vi "Delete Config.vi"(8 "error in (no error)":errorcluster, 9 "Config Selected":string, 10 "Config Select Ref":refnum<vi>, 11 "GUI in":refnum<class "GUI.lvclass">) -> (0 "error out":errorcluster, 3 "GUI out":refnum<class "GUI.lvclass">)   [LabVIEW 2020, in "GUI.lvlib" / "GUI.lvclass"]
uses:
  GUI.lvclass
  GUI.lvclass/GUI.ctl
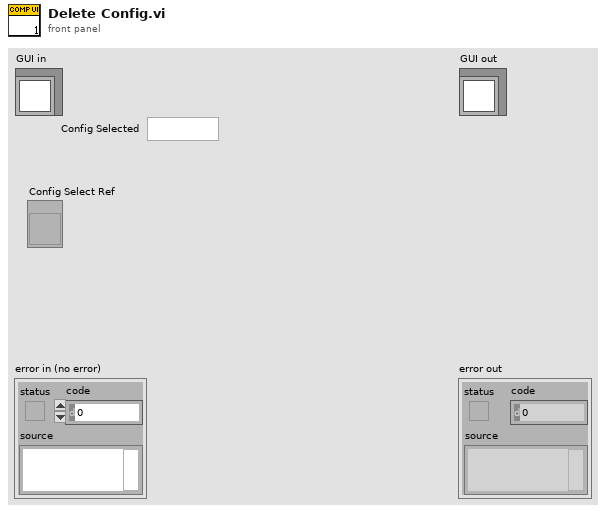
[diagram p1: front panel]
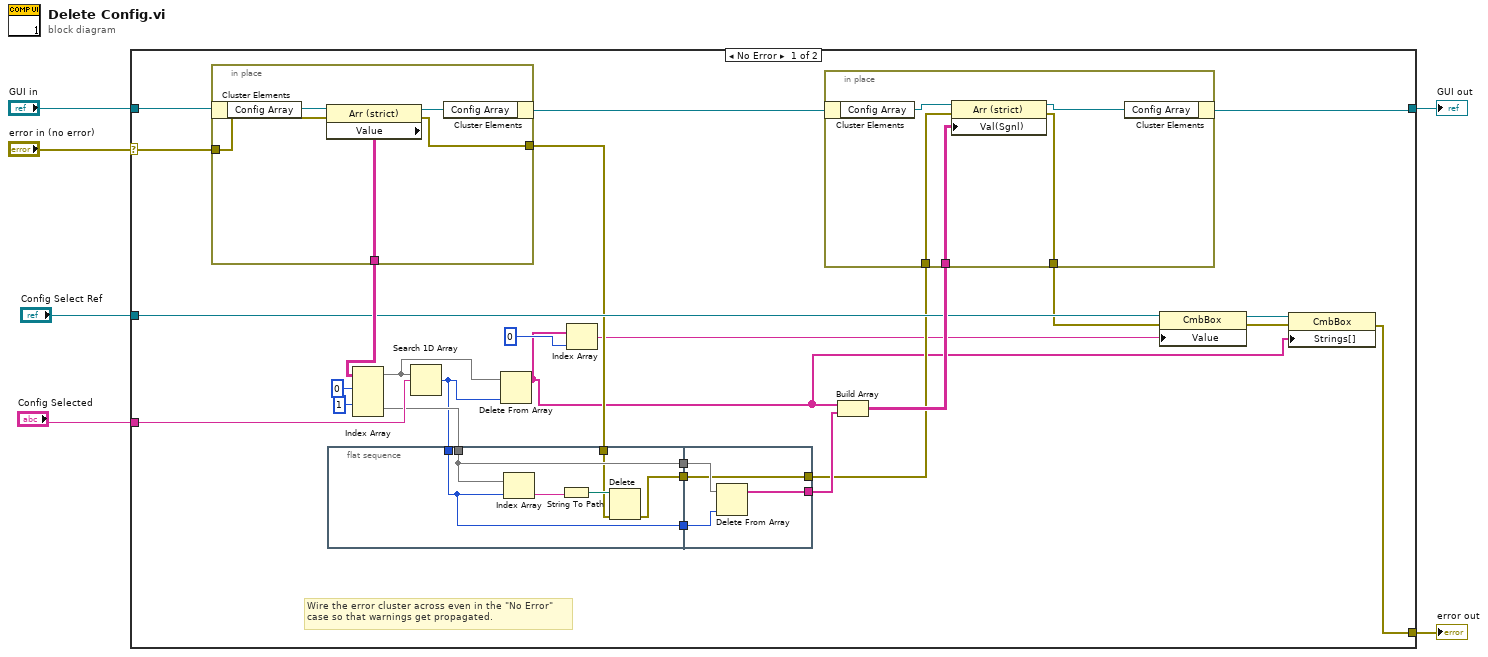
[diagram p0: block diagram]
diagram:
  n1 = case shown="No Error" "error in (no error)" {
    selector: "error in (no error)" -> [w18 w54]
    tunnel: [w9 w54] -> w5
    tunnel: [w21 w53] -> w3
    tunnel: "GUI in" -> [w32 w53]
    tunnel: "Config Selected" -> [w28 _]
    tunnel: "Config Select Ref" -> [w19 _]
    frame No Error {
      # "Wire the error cluster across even in the \"No Error\"\ncase so that warnings get propagated."
      n2 = in-place {
        in-place-border: [w51] -> w29
        in-place-border: w18 -> [w49]
        in-place-border: [w48] -> w17
        n3 = in-place-cluster #1(w32) -> ("Config Array"=w52:refnum<vi>)
        n4 = property class="Arr (strict)"(reference=w52, error in=w49) -> (reference out=w50:refnum<vi>, error out=w48:errorcluster, "Value"=w51:string[][])
        n5 = in-place-cluster #1("Config Array"=w50) -> (w22:refnum<class "GUI.lvclass">)
      }
      n6 = flat-sequence {
        tunnel: w26 -> [w41]
        tunnel: w7 -> [w40]
        tunnel: [w41] -> w25
        tunnel: [w40] -> w24
        tunnel: w17 -> [w39]
        tunnel: [w38] -> w16
        tunnel: w25 -> [w47]
        tunnel: w24 -> [w46]
        tunnel: [w45] -> w23
        tunnel: [w44] -> w15
        tunnel: w16 -> [w44]
        frame #0 {
          n7 = Index Array(array=w41, index=w40) -> (element=w43:string)
          n8 = String To Path(string=w43) -> (path=w42:path)
          n9 = Delete(path (use dialog)=w42, error in=w39) -> (error out=w38:errorcluster)  [unwired: 3 in, 2 out]
        }
        frame #1 {
          n10 = Delete From Array(array=w47, index=w46) -> (array with subset deleted=w45:string[])  [unwired: 1 in, 1 out]
        }
      }
      n11 = Index Array(array=w29, index (row) #1=0 ("index (row)"), index (row) #2=1 ("index (row)")) -> (element #1=w27:string[], element #2=w26:string[])  [unwired: 2 in]
      n12 = Search 1D Array(1D array=w27, element=w28) -> (index of element=w7:i32)  [unwired: 1 in]
      n13 = Delete From Array(array=w27, index=w7) -> (array with subset deleted=w8:string[])  [unwired: 1 in, 1 out]
      n14 = Index Array(array=w8, index=0) -> (element=w12:string)
      n15 = Build Array(w8, w23) -> (w20:string[][])
      n16 = in-place {
        in-place-border: w20 -> [w35]
        in-place-border: w15 -> [w34]
        in-place-border: [w33] -> w14
        n17 = in-place-cluster #2(w22) -> ("Config Array"=w37:refnum<vi>)
        n18 = property class="Arr (strict)"(reference=w37, error in=w34, "Val(Sgnl)"=w35) -> (reference out=w36:refnum<vi>, error out=w33:errorcluster)
        n19 = in-place-cluster #2("Config Array"=w36) -> (w21:refnum<class "GUI.lvclass">)
      }
      n20 = property class="CmbBox"(reference=w19, error in=w14, "Value"=w12) -> (reference out=w11:refnum<vi>, error out=w10:errorcluster)
      n21 = property class="CmbBox"(reference=w11, error in=w10, "Strings[]"=w8) -> (error out=w9:errorcluster)  [unwired: 1 out]
    }
    frame Error {
    }
  }
  "error out" <- w5
  "GUI out" <- w3
